vi "Get Triangle Index.vi"(9 "Y Dimension":i32, 11 "X Dimension":i32) -> (3 "Triangle Index Array":u32[](array[numeric]))   [LabVIEW 2020, in "3D Plot Datatype.lvclass"]
uses:
  <vilib>/Math Plots/3D Math Plots/3D Plot/3D Plot Datatype/3D Plot Datatype.lvclass
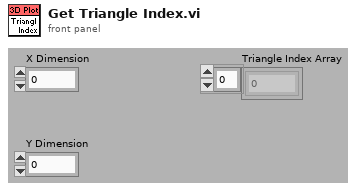
[diagram p1: front panel]
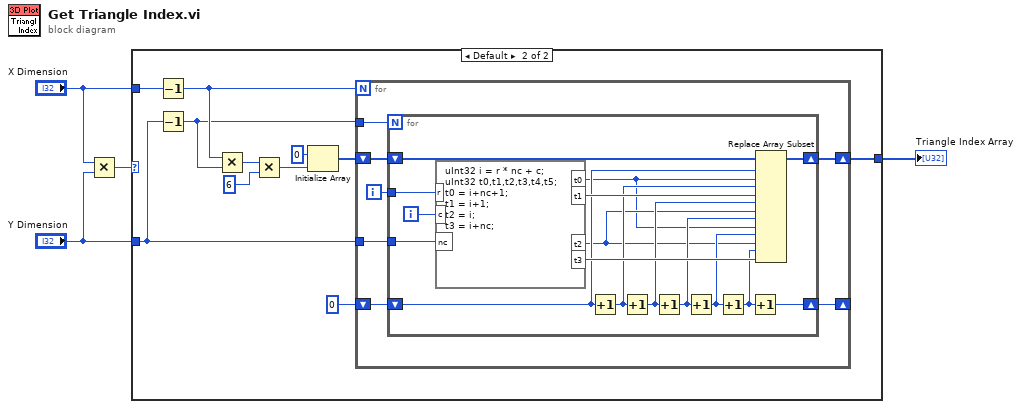
[diagram p0: block diagram]
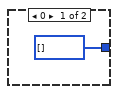
[diagram p2: hidden frame]
diagram:
  n1 = Multiply(x="X Dimension", y="Y Dimension") -> (x*y=w3:i32)
  n2 = case shown="Default" w3 {
    tunnel: "X Dimension" -> [_ w16]
    tunnel: "Y Dimension" -> [_ w15]
    tunnel: [u32[] [] w14] -> w4
    frame 0 {
    }
    frame Default {
      n3 = Decrement(x=w16) -> (x-1=w9:i32)
      n4 = Decrement(x=w15) -> (x-1=w8:i32)
      n5 = Multiply(x=w9, y=w8) -> (x*y=w12:i32)
      n6 = Multiply(x=w12, y=6) -> (x*y=w10:i32)
      n7 = Initialize Array(u32 0, w10) -> (w7:u32[])
      n8 = for {
        N: w9 -> [_]
        shift-right: [w19] -> w14
        shift-left: w7 -> [w23]
        tunnel: w8 -> [w21]
        tunnel: w15 -> [w20]
        shift-right: [w18] -> _
        shift-left: 0 -> [w17]
        i -> [w22]
        n9 = for {
          N: w21 -> [_]
          tunnel: w22 -> [w37]
          tunnel: w20 -> [w35]
          shift-right: [w38] -> w19
          shift-left: w23 -> [w39]
          shift-right: [w34] -> w18
          shift-left: w17 -> [w26]
          i -> [w36]
          n10 = formula code="uInt32 i = r * nc + c; \nuInt32 t0,t1,t2,t3,t4,t5;\nt0 = i+nc+1; \nt1 = i+1; \nt2 = i; \nt3 = i+nc;"("r"=w37, "nc"=w35, "c"=w36) -> ("t0"=w24:u32, "t1"=w33:u32, "t2"=w25:u32, "t3"=w32:u32)
          n11 = Increment(x=w26) -> (x+1=w27:i32)
          n12 = Increment(x=w27) -> (x+1=w28:i32)
          n13 = Increment(x=w28) -> (x+1=w29:i32)
          n14 = Increment(x=w29) -> (x+1=w30:i32)
          n15 = Increment(x=w30) -> (x+1=w31:i32)
          n16 = Increment(x=w31) -> (x+1=w34:i32)
          n17 = Replace Array Subset(array=w39, new element #1=w24, index #1=w26, new element #2=w33, index #2=w27, new element #3=w25, index #3=w28, new element #4=w24, index #4=w29, new element #5=w25, index #5=w30, new element #6=w32, index #6=w31) -> (w38:u32[])
        }
      }
    }
  }
  "Triangle Index Array" <- w4
